vi "read_corr_coeff.vi"() -> (0 "bck: a\n(ax+b)":dbl=465.88005, 1 "bck: b\n(ax+b)":dbl=465.88005, 2 "A\n(Ax^2+Bx+C)":dbl, 3 "B\n(Ax^2+Bx+C)":dbl, 4 "C\n(Ax^2+Bx+C)":dbl)   [LabVIEW 2022 SP3]
panel:
  out "additional info 16":string
  out "string":string
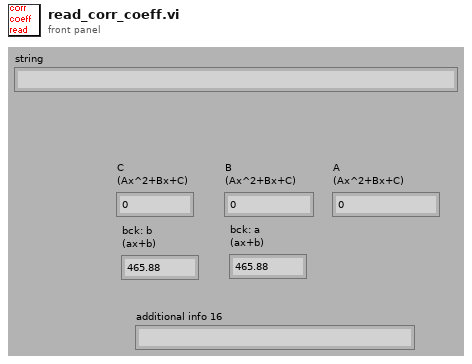
[diagram p1: front panel]
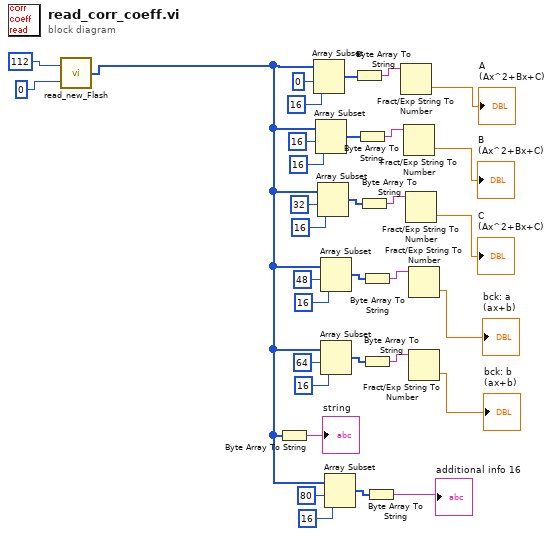
[diagram p0: block diagram]
diagram:
  n1 = call "read_new_Flash.vi"("address (3 bytes)"=u32 0, "read_bytes"=u64 112) -> ("Read_data"=w2:u8[])
  n2 = Byte Array To String(unsigned byte array=w2) -> (string=→"string":string)
  n3 = Array Subset(array=w2, index=0, length=16) -> (w27:u8[])
  n4 = Array Subset(array=w2, index=16, length=16) -> (w23:u8[])
  n5 = Array Subset(array=w2, index=32, length=16) -> (w20:u8[])
  n6 = Array Subset(array=w2, index=48, length=16) -> (w14:u8[])
  n7 = Array Subset(array=w2, index=64, length=16) -> (w9:u8[])
  n8 = Array Subset(array=w2, index=80, length=16) -> (w3:u8[])
  n9 = Byte Array To String(unsigned byte array=w27) -> (string=w26:string)
  n10 = Byte Array To String(unsigned byte array=w23) -> (string=w24:string)
  n11 = Byte Array To String(unsigned byte array=w20) -> (string=w21:string)
  n12 = Byte Array To String(unsigned byte array=w14) -> (string=w15:string)
  n13 = Byte Array To String(unsigned byte array=w9) -> (string=w10:string)
  n14 = Byte Array To String(unsigned byte array=w3) -> (string=→"additional info 16":string)
  n15 = Fract/Exp String To Number(string=w26) -> (number=→"A\n(Ax^2+Bx+C)":dbl)  [unwired: 3 in, 1 out]
  n16 = Fract/Exp String To Number(string=w24) -> (number=→"B\n(Ax^2+Bx+C)":dbl)  [unwired: 3 in, 1 out]
  n17 = Fract/Exp String To Number(string=w21) -> (number=→"C\n(Ax^2+Bx+C)":dbl)  [unwired: 3 in, 1 out]
  n18 = Fract/Exp String To Number(string=w15) -> (number=→"bck: a\n(ax+b)":dbl)  [unwired: 3 in, 1 out]
  n19 = Fract/Exp String To Number(string=w10) -> (number=→"bck: b\n(ax+b)":dbl)  [unwired: 3 in, 1 out]
